vi "WDT Find First Error and Warning.vi"(4 "error in (no error)":errorcluster, 7 "Error Codes":i32[](array[numeric])) -> (0 "error out":errorcluster, 3 "error?":bool)   [LabVIEW 2020]
doc: "Find the first error or warning in the input error codes or error in cluster."
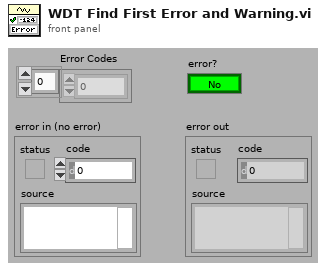
[diagram p1: front panel]
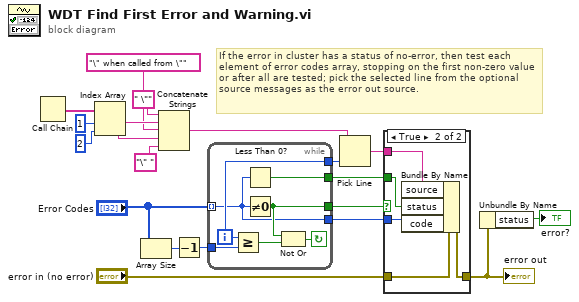
[diagram p0: block diagram]
diagram:
  # "If the error in cluster has a status of no-error, then test each element of error codes array, stopping on the first non-zero value or after all are tested; pick the selected line from the optional source messages as the error out source."
  n1 = Call Chain() -> (call chain=w15:string[])
  n2 = Index Array(array=w15, index #1=1 ("Index"), index #2=2 ("Index")) -> (element #1=w17:string, element #2=w14:string)
  n3 = Array Size(array="Error Codes") -> (size(s)=w8:i32)
  n4 = Concatenate Strings(" \"" ("Substring"), w17, "\" when called from \"", w14, "\" ") -> (w16:string)
  n5 = Decrement(x=w8) -> (x-1=w9:i32)
  n6 = while {
    tunnel: [w21] -> w4
    tunnel: w9 -> [w23]
    tunnel: "Error Codes" -> [w22] mode=indexing
    tunnel: [w24] -> w10
    tunnel: [w25] -> w5
    tunnel: [w22] -> w7
    i -> [w24]
    stop <- w26 continue-if-true
    n7 = Greater Or Equal?(x=w24, y=w23) -> (x >= y?=w27:bool)
    n8 = Less Than 0?(x=w22) -> (x < 0?=w21:bool)
    n9 = Not Equal To 0?(x=w22) -> (x != 0?=w25:bool)
    n10 = Not Or(1:w27, 2:w25) -> (0:w26:bool)
  }
  n11 = Pick Line(multi-line string=w16, line index=w10) -> (output string=w6:string)  [unwired: 1 out]
  n12 = case shown="True" w5 {
    tunnel: [w28 w33] -> w2
    tunnel: w7 -> [_ w32]
    tunnel: w6 -> [_ w29]
    tunnel: w4 -> [_ w30]
    tunnel: "error in (no error)" -> [w28 w31]
    frame False {
    }
    frame True {
      n13 = Bundle By Name(cluster=w31, "source"=w29, "status"=w30, "code"=w32) -> (w33:errorcluster)
    }
  }
  "error out" <- w2
  n14 = Unbundle By Name(w2) -> ("status"=→"error?":bool)
